vi "LvMPDC_CMD_seek.vi"(6 "timeout_ms":i32=25000, 7 "time pos":dbl, 8 "error in (no error)":errorcluster, 9 "ReadBytes":i32=1024, 10 "song pos":i32, 11 "Connect ID":refnum<k5>) -> (0 "error out":errorcluster, 3 "Connect ID out":refnum<k5>)   [LabVIEW 2012]
panel:
  # "LvMPDC:: CMD seek"
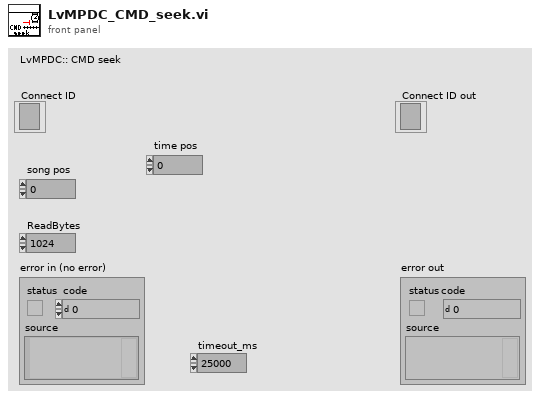
[diagram p1: front panel]
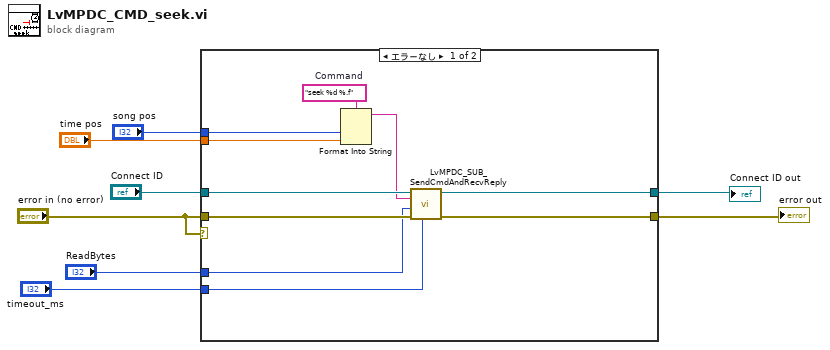
[diagram p0: block diagram]
diagram:
  n1 = case shown="エラーなし" "error in (no error)" {
    tunnel: "Connect ID" -> [w16 w20]
    tunnel: "error in (no error)" -> [w18 w19]
    tunnel: [w15 w20] -> w7
    tunnel: [w17 w19] -> w6
    tunnel: "timeout_ms" -> [w13 _]
    tunnel: "ReadBytes" -> [w14 _]
    tunnel: "song pos" -> [w12 _]
    tunnel: "time pos" -> [w9 _]
    frame No Error {
      w11 = "seek %d %.f"  # Command
      n2 = Format Into String(format string=w11, w12, w9) -> (resulting string=w10:string)  [unwired: 2 in, 1 out]
      n3 = call "LvMPDC_SUB_SendCmdAndRecvReply.vi"("timeout_ms"=w13, "error in (no error)"=w18, "ReadBytes"=w14, "Command"=w10, "Connect ID"=w16) -> ("error out"=w17:errorcluster, "Connect ID out"=w15:refnum<k5>)  [unwired: 4 in, 1 out]
    }
    frame Error {
    }
  }
  "Connect ID out" <- w7
  "error out" <- w6
